vi "Decode VSS Simulator Package.vi"(5 "Version":string(combo)="Auto", 8 "error in (no error)":errorcluster, 10 "unsigned byte array 2":u8[](array[numeric]), 11 "unsigned byte array":u8[](array[numeric])) -> (2 "Field Size out":T1={"field_length"=1500, "field_width"=1300, "goal_width"=400, "goal_depth"=100, "center_circle_radius"=200, "defense_width"=700, "defense_depth"=150, "free_kick_from_defense_dist"=375, "penalty_spot_from_field_line_dist"=375, "penalty_line_from_spot_dist"=0, "half_moon_depth"=50, "half_moon_width"=200}, 3 "Detection Frame":T2 {"robots_blue"."height" format="%+4.3f"; "robots_blue"."pixel_y" format="%+4.3f"; "robots_blue"."pixel_x" format="%+4.3f"; "robots_blue"."orientation" format="%+4.3f"; "robots_blue"."y" format="%+4.3f"; "robots_blue"."confidence" format="%4.3f"; "robots_blue"."x" format="%+4.3f"; "robots_yellow"."height" format="%+4.3f"; "robots_yellow"."pixel_y" format="%+4.3f"; "robots_yellow"."pixel_x" format="%+4.3f"; "robots_yellow"."orientation" format="%+4.3f"; "robots_yellow"."y" format="%+4.3f"; "robots_yellow"."confidence" format="%4.3f"; "robots_yellow"."x" format="%+4.3f"})   [LabVIEW 2017]
uses:
  VSS Detection Frame.ctl
  SSL Detection Robot.ctl
  <vilib>/Analysis/Matrix/Datatypes/RealMatrix.ctl
  SSL Detection Ball.ctl
  VSS Geometry Field Size.ctl
  <vilib>/Analysis/Matrix/NI_Matrix.lvlib
panel:
  in  "Field Size in":T1={"field_length"=1500, "field_width"=1300, "goal_width"=400, "goal_depth"=100, "center_circle_radius"=200, "defense_width"=700, "defense_depth"=150, "free_kick_from_defense_dist"=375, "penalty_spot_from_field_line_dist"=375, "penalty_line_from_spot_dist"=0, "half_moon_depth"=50, "half_moon_width"=200}
  out "error out":errorcluster
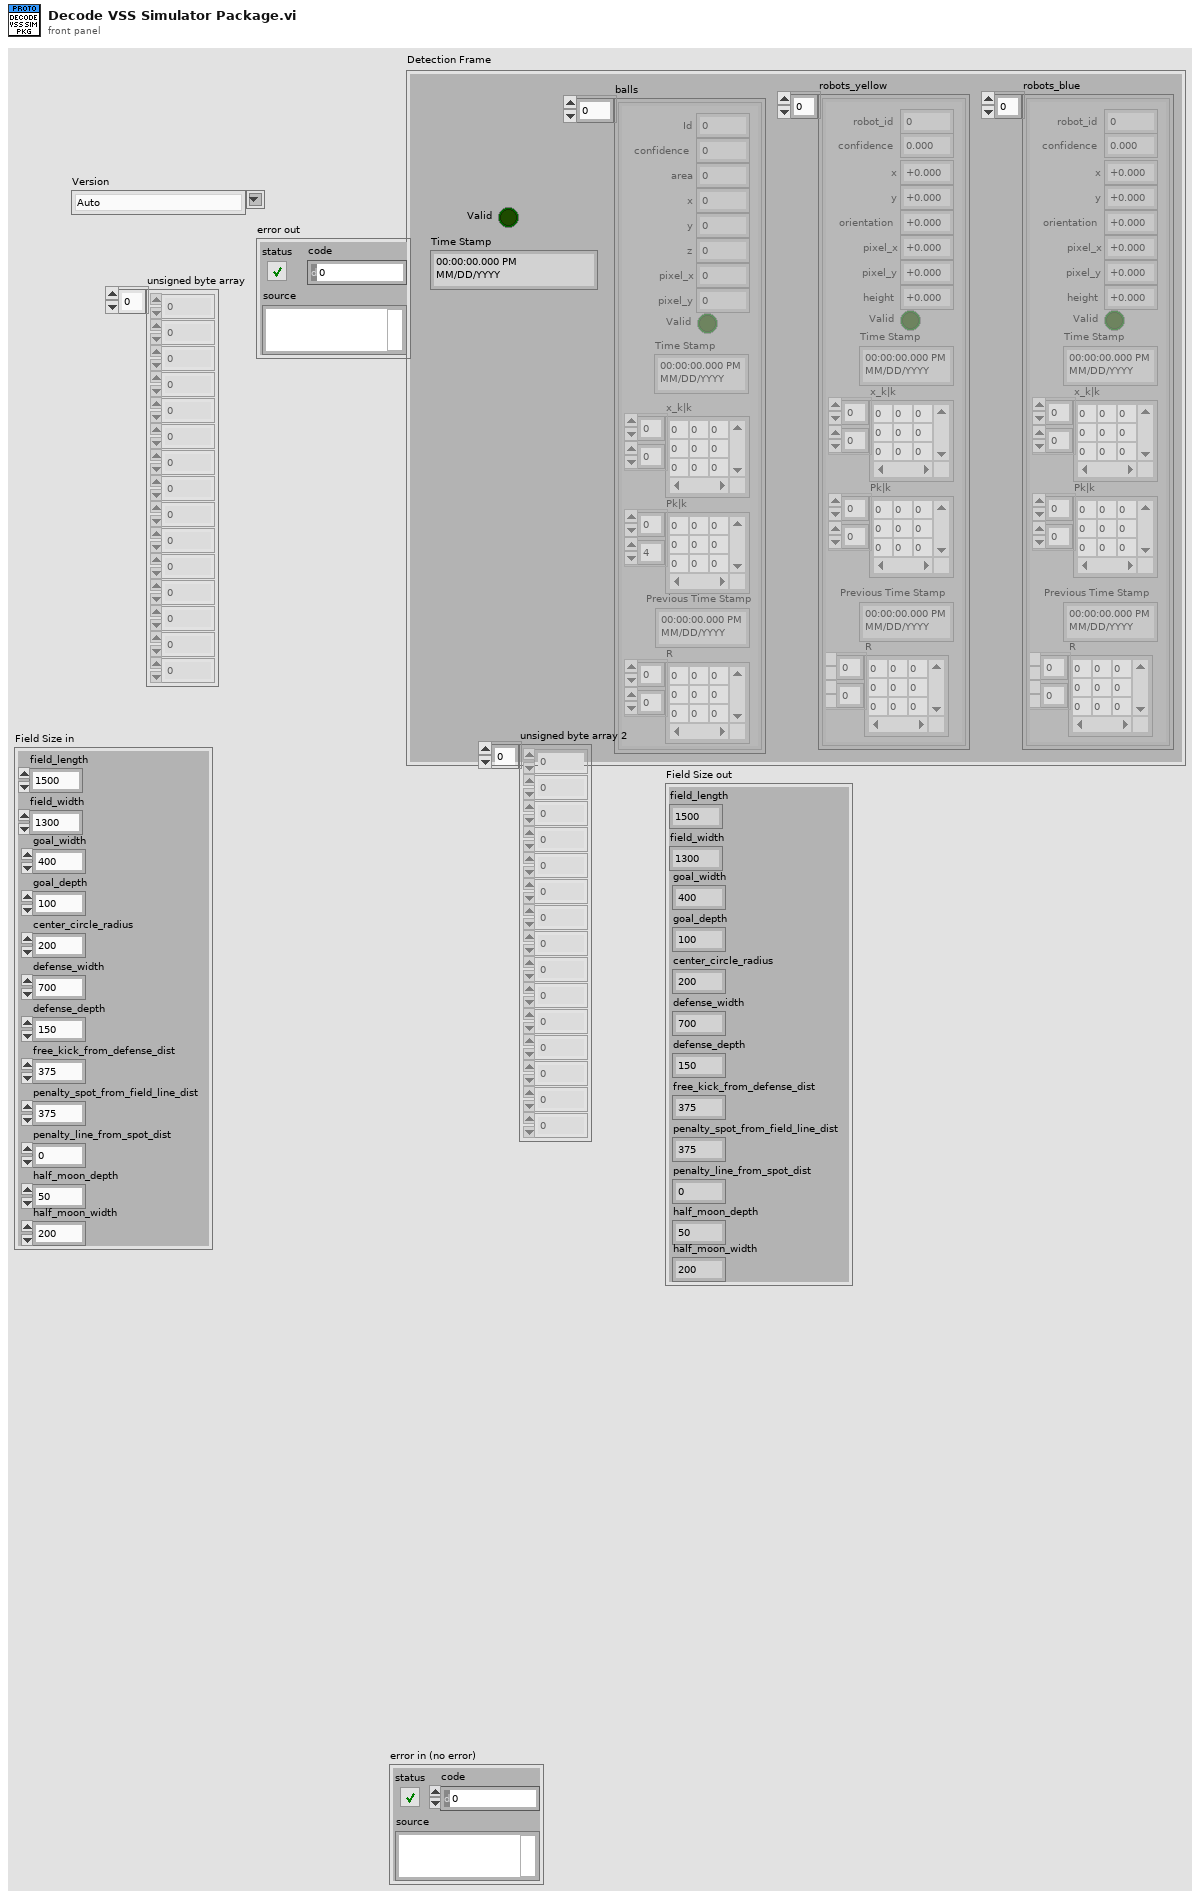
[diagram p1: front panel]
types:
  T1 = typedef "VSS Geometry Field Size.ctl" = cluster{"field_length":u32, "field_width":u32, "goal_width":u32, "goal_depth":u32, "center_circle_radius":u32, "defense_width":u32, "defense_depth":u32, "free_kick_from_defense_dist":u32, "penalty_spot_from_field_line_dist":u32, "penalty_line_from_spot_dist":u32, "half_moon_depth":u32, "half_moon_width":u32}
  T2 = typedef "VSS Detection Frame.ctl" = cluster{"robots_yellow":T3[], "robots_blue":T3[], "balls":T5[], "Valid":bool, "Time Stamp":timestamp}
  T3 = typedef "SSL Detection Robot.ctl" = cluster{"x":sgl, "robot_id":u32, "confidence":sgl, "y":sgl, "orientation":sgl, "pixel_x":sgl, "pixel_y":sgl, "height":sgl, "Valid":bool, "Time Stamp":timestamp, "x_k|k":T4, "Pk|k":T4, "Previous Time Stamp":timestamp, "R":T4}
  T4 = typedef "NI_Matrix.lvlib/RealMatrix.ctl" = dbl[][]
  T5 = typedef "SSL Detection Ball.ctl" = cluster{"x":sgl, "area":u32, "confidence":sgl, "y":sgl, "z":sgl, "pixel_x":sgl, "pixel_y":sgl, "Valid":bool, "Time Stamp":timestamp, "x_k|k":T4, "Pk|k":T4, "Id":u32, "Previous Time Stamp":timestamp, "R":T4}
  T6 = typedef "SSL Detection Frame.ctl" = cluster{"robots_yellow":T3[], "robots_blue":T3[], "balls":T5[], "Valid":bool, "Time Stamp":timestamp}
  T7 = typedef "SSL Geometry Camera Calibration.ctl" = cluster{"camera_id":u32, "focal_length":sgl, "principal_point_x":sgl, "principal_point_y":sgl, "distortion":sgl, "q0":sgl, "q1":sgl, "q2":sgl, "q3":sgl, "tx":sgl, "ty":sgl, "tz":sgl, "derived_camera_world_tx":sgl, "derived_camera_world_ty":sgl, "derived_camera_world_tz":sgl}
  T8 = cluster{"line_width":u32, "field_length":u32, "field_width":u32, "boundary_width":u32, "referee_width":u32, "goal_width":u32, "goal_depth":u32, "goal_wall_width":u32, "center_circle_radius":u32, "defense_radius":u32, "defense_stretch":u32, "free_kick_from_defense_dist":u32, "penalty_spot_from_field_line_dist":u32, "penalty_line_from_spot_dist":u32}
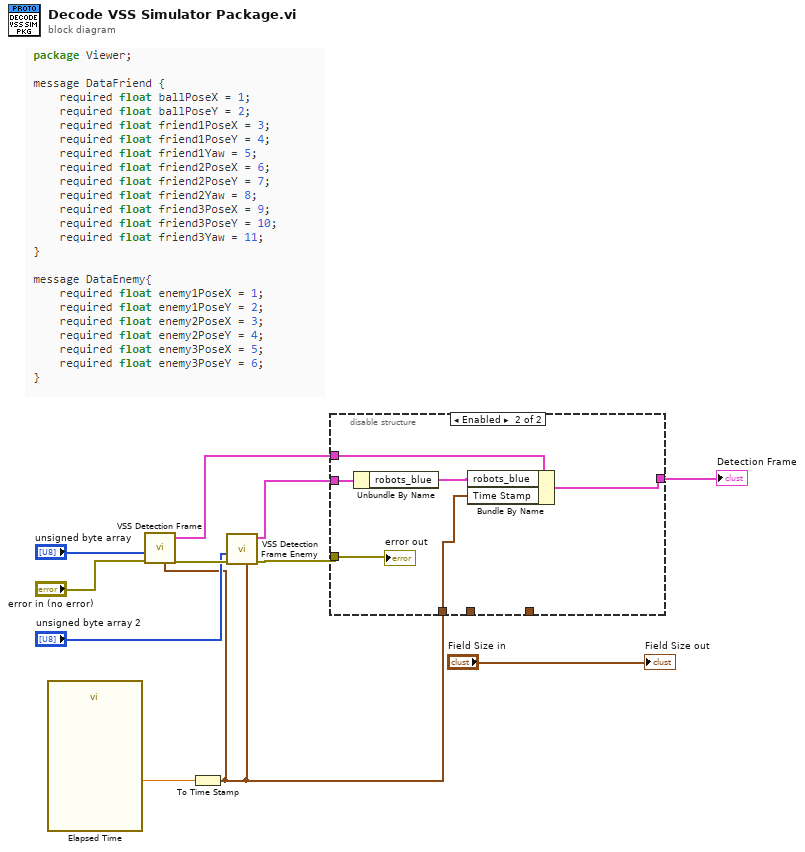
[diagram p0: block diagram]
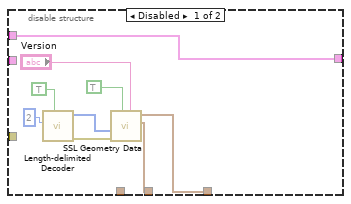
[diagram p2: hidden frame]
diagram:
  n1 = call "Elapsed Time"() -> ("Elapsed Time (s)"=w2:dbl)  [unwired: 12 in, 7 out]
  n2 = To Time Stamp(1:w2) -> (0:w1:timestamp)
  n3 = call "VSS Detection Frame.vi"("time stamp"=w1, "error in"="error in (no error)", "Array"="unsigned byte array") -> ("error out"=w6:errorcluster, "Detection Frame"=w11:T6)  [unwired: 6 in, 1 out]
  n4 = call "VSS Detection Frame Enemy.vi"("time stamp"=w1, "error in"=w6, "Array"="unsigned byte array 2") -> ("error out"=w5:errorcluster, "Detection Frame"=w8:T6)  [unwired: 7 in]
  n5 = disable-structure shown="Enabled" {
    disable-tunnel: w11 -> [w14 w28]
    disable-tunnel: w8 -> [_ w25]
    disable-tunnel: [w14 w27] -> w7
    disable-tunnel: w5 -> [_ w26]
    disable-tunnel: [w13 _] -> _
    disable-tunnel: [w12 _] -> _
    disable-tunnel: w1 -> [_ w23]
    frame Disabled {
      n6 = call "Length-delimited Decoder.vi"("Optional"=TRUE, "Key"=2) -> ("error out"=w18:errorcluster, "Length-delimited"=w20:u8[], "error in (no error)"=w17:errorcluster)  [unwired: 5 in, 2 out]
      n7 = call "SSL Geometry Data.vi"("Version"="Version", "Optional"=TRUE, "error in"=w18, "Array"=w20) -> ("error out"=w22:errorcluster, "Geometry Camera Calibration"=w12:T7, "Field Size"=w13:T8)  [unwired: 5 in]
    }
    frame Enabled {
      n8 = Unbundle By Name(w25) -> ("robots_blue"=w24:T3[])
      n9 = Bundle By Name(cluster=w28, "robots_blue"=w24, "Time Stamp"=w23) -> (w27:T6)
      "error out" <- w26
    }
  }
  "Detection Frame" <- w7
  "Field Size out" <- "Field Size in"
